vi "Prepare Paths For Expiration Check.vi"(0 "SG Path Group in":refnum<class "SG Path Group.lvclass">, 5 "TSM Context":T1, 11 "error in":errorcluster) -> (4 "SG Path Group out":refnum<class "SG Path Group.lvclass">, 15 "error out":errorcluster)   [LabVIEW 2023, in "RFFixtureCharact.PXI.lvlib" / "SG Path Group.lvclass"]
uses:
  SG Path Group.lvclass
  SG Path Group.lvclass/SG Path Group.ctl
  <vilib>/NI_TestStand_SemiconductorModule/NI_TestStand_Semiconductor_Module.lvlibp
  Common/Base Classes/Path Group/Path Group.lvclass
  <vilib>/addons/_RFCalAndCharactDatabase/NI_RFCalAndCharact_Database_API.lvlibp/Characterization/Characterization.lvlib
  Common/Base Classes/Path/Path.lvclass
  <vilib>/NI_TestStand_SemiconductorModule/NI_TestStand_Semiconductor_Module.lvlibp/PinMap/RF/RFSG/PinToNIRFSGSession.vi
  Public/Charact Result Accessor/Scalar/Scalar Charact Result Accessor.lvclass
  C:/rfcal/AuxTools/STSRFFixtureCharactUtility/Source/Code Modules/Fixture/Public/Charact Result Accessor/Base/Charact Result Accessor.lvclass
  C:/rfcal/AuxTools/STSRFFixtureCharactUtility/Source/Code Modules/Common/Result Accessor/Result Accessor.lvclass
  C:/rfcal/AuxTools/STSRFFixtureCharactUtility/Source/Code Modules/Fixture/Public/Charact Result Accessor/Scalar/Scalar Charact Result Accessor.lvclass
  <vilib>/NI_TestStand_SemiconductorModule/NI_TestStand_Semiconductor_Module.lvlibp/PinMap/General/SemiconductorModuleContext.ctl
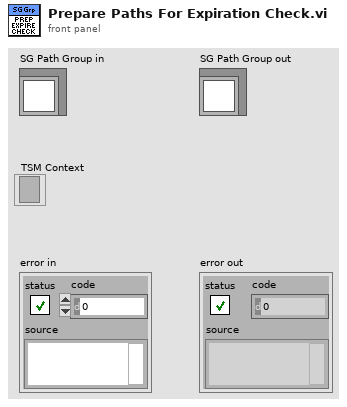
[diagram p1: front panel]
types:
  T1 = typedef "NI_TestStand_Semiconductor_Module.lvlibp/SemiconductorModuleContext.ctl" = refnum<k7>
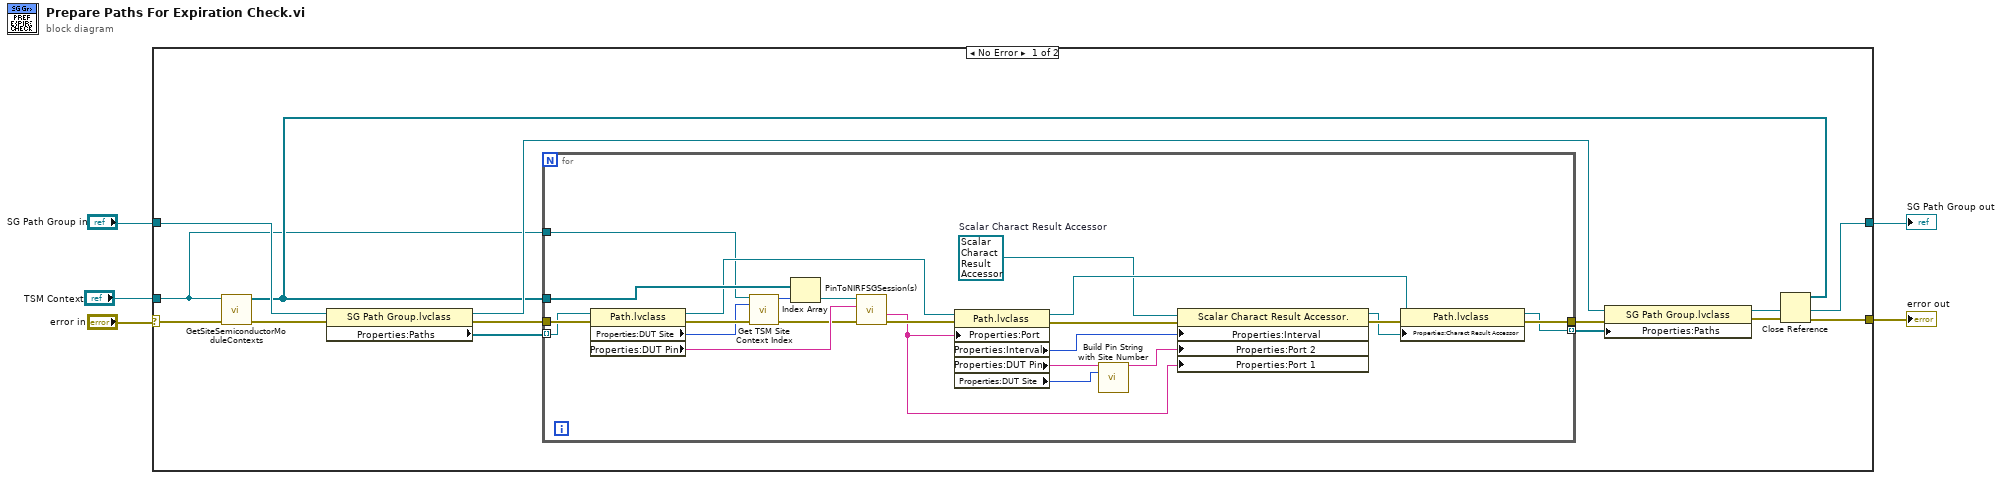
[diagram p0: block diagram]
diagram:
  n1 = case shown="No Error" "error in" {
    selector: "error in" -> [w7 w44]
    tunnel: "TSM Context" -> [w6 _]
    tunnel: "SG Path Group in" -> [w10 w43]
    tunnel: [w9 w44] -> w1
    tunnel: [w11 w43] -> w2
    frame No Error {
      n2 = call <vilib>:"GetSiteSemiconductorModuleContexts.vi"("error in (no error)"=w7, "Semiconductor Module Context"=w6) -> ("error out"=w15:errorcluster, "Site Semiconductor Module Contexts"=w8:T1[])  [unwired: 8 in]
      n3 = property class="SG Path Group.lvclass"(reference=w10, error in=w15) -> (reference out=w13:refnum<class "SG Path Group.lvclass">, error out=w17:errorcluster, "Properties:Paths"=w16:refnum<class "Path.lvclass">[])
      n4 = for {
        tunnel: w17 -> [w37]
        tunnel: w8 -> [w42]
        tunnel: [w28] -> w18
        tunnel: w16 -> [w36] mode=indexing
        tunnel: [w25] -> w12 mode=indexing
        tunnel: w6 -> [w31]
        w21 = refnum<class "Scalar Charact Result Accessor.lvclass"> refnum  # Scalar Charact Result Accessor
        n5 = property class="Path.lvclass"(reference=w36, error in=w37) -> (reference out=w38:refnum<class "Path.lvclass">, error out=w40:errorcluster, "Properties:DUT Site"=w33:i32, "Properties:DUT Pin"=w35:string)
        n6 = call "Get TSM Site Context Index.vi"("Semiconductor Module Context"=w31, "Site Number"=w33, "error in (no error)"=w40) -> ("index of Site TSM Context"=w32:i32, "error out"=w34:errorcluster)  [unwired: 11 in]
        n7 = Index Array(array=w42, index=w32) -> (element=w41:T1)
        n8 = call-poly <vilib>:"PinToNIRFSGSession(s).vi"("error in (no error)"=w34, "Pin"=w35, "Semiconductor Module Context"=w41) -> ("error out"=w39:errorcluster, "Port"=w30:string)  [unwired: 4 in, 3 out]
        n9 = property class="Path.lvclass"(reference=w38, error in=w39, "Properties:Port"=w30) -> (reference out=w26:refnum<class "Path.lvclass">, error out=w22:errorcluster, "Properties:Interval"=w19:i32, "Properties:DUT Pin"=w23:string, "Properties:DUT Site"=w24:i32)
        n10 = call <vilib>:"Build Pin String with Site Number.vi"("Pin Name"=w23, "Site Number"=w24) -> ("Pin String"=w20:string)  [unwired: 13 in]
        n11 = property class="Scalar Charact Result Accessor."(reference=w21, error in=w22, "Properties:Interval"=w19, "Properties:Port 2"=w20, "Properties:Port 1"=w30) -> (reference out=w27:refnum<class "Scalar Charact Result Accessor.lvclass">, error out=w29:errorcluster)
        n12 = property class="Path.lvclass"(reference=w26, error in=w29, "Properties:Charact Result Accessor"=w27) -> (reference out=w25:refnum<class "Path.lvclass">, error out=w28:errorcluster)
      }
      n13 = property class="SG Path Group.lvclass"(reference=w13, error in=w18, "Properties:Paths"=w12) -> (reference out=w11:refnum<class "SG Path Group.lvclass">, error out=w14:errorcluster)
      n14 = Close Reference(reference=w8, error in (no error)=w14) -> (error out=w9:errorcluster)
    }
    frame Error {
    }
  }
  "error out" <- w1
  "SG Path Group out" <- w2
